vi "nome_arquivo_adq.vi"(0 "caminho":path, 7 "JW":string, 9 "JK":string, 11 "JG":string) -> (4 "resulting string":string)   [LabVIEW 2019]
doc: "VI de criação do nome do arquivo que será salvo, utilizando as velocidades do líquido e a configuração atual."
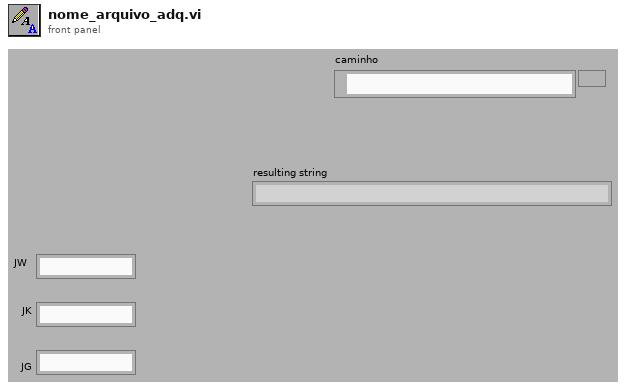
[diagram p1: front panel]
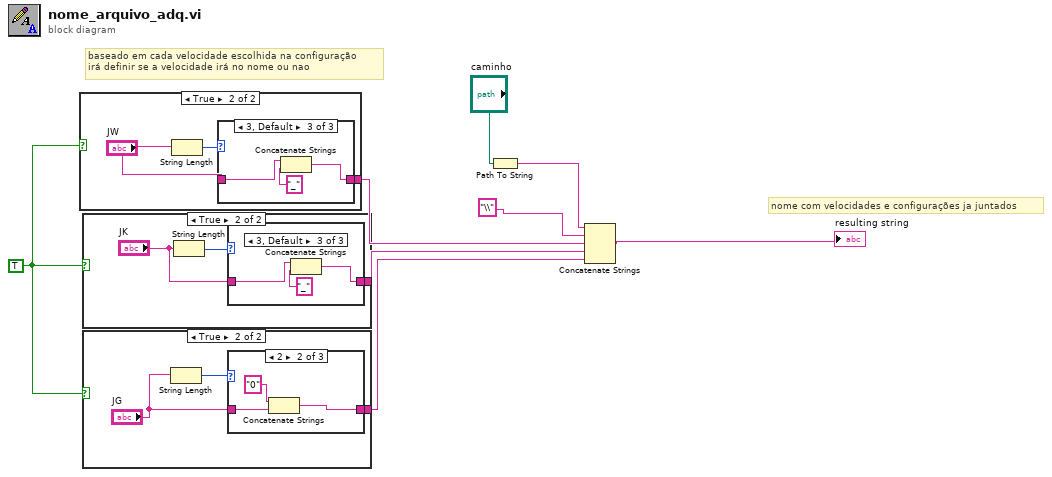
[diagram p0: block diagram]
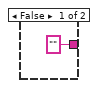
[diagram p2: hidden frame]
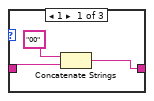
[diagram p3: hidden frame]
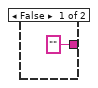
[diagram p5: hidden frame]
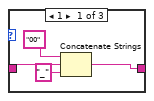
[diagram p6: hidden frame]
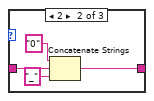
[diagram p7: hidden frame]
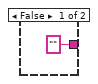
[diagram p8: hidden frame]
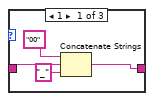
[diagram p9: hidden frame]
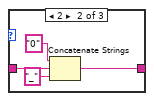
[diagram p10: hidden frame]
diagram:
  w1 = TRUE
  # "nome com velocidades e configurações ja juntados"
  # "baseado em cada velocidade escolhida na configuração\nirá definir se a velocidade irá no nome ou nao"
  n1 = case shown="True" w1 {
    tunnel: ["" w10] -> w7
    frame False {
    }
    frame True {
      n2 = String Length(string="JW") -> (length=w12:i32)
      n3 = case shown="3, Default" w12 {
        tunnel: "JW" -> [w15 w19 w23]
        tunnel: [w16 w18 w21] -> w10
        frame 1 {
          n4 = Concatenate Strings("00" ("string"), w15, "_" ("string")) -> (w16:string)
        }
        frame 2 {
          n5 = Concatenate Strings("0" ("string"), w19, "_" ("string")) -> (w18:string)
        }
        frame 3, Default {
          n6 = Concatenate Strings(w23, "_" ("string")) -> (w21:string)
        }
      }
    }
  }
  n7 = case shown="True" w1 {
    tunnel: ["" w25] -> w6
    frame False {
    }
    frame True {
      n8 = String Length(string="JK") -> (length=w27:i32)
      n9 = case shown="3, Default" w27 {
        tunnel: "JK" -> [w30 w34 w38]
        tunnel: [w31 w33 w36] -> w25
        frame 1 {
          n10 = Concatenate Strings("00" ("string"), w30, "_" ("string")) -> (w31:string)
        }
        frame 2 {
          n11 = Concatenate Strings("0" ("string"), w34, "_" ("string")) -> (w33:string)
        }
        frame 3, Default {
          n12 = Concatenate Strings(w38, "_" ("string")) -> (w36:string)
        }
      }
    }
  }
  n13 = case shown="True" w1 {
    tunnel: ["" w42] -> w5
    frame False {
    }
    frame True {
      n14 = String Length(string="JG") -> (length=w41:i32)
      n15 = case shown="2" w41 {
        tunnel: "JG" -> [w44 w47 w49]
        tunnel: [w45 w46 w49] -> w42
        frame 1 {
          n16 = Concatenate Strings("00" ("string"), w44) -> (w45:string)
        }
        frame 2 {
          n17 = Concatenate Strings("0" ("string"), w47) -> (w46:string)
        }
        frame 3, Default {
        }
      }
    }
  }
  n18 = Path To String(path="caminho") -> (string=w3:string)
  n19 = Concatenate Strings(w3, "\\", w7, w6, w5) -> (→"resulting string":string)
